vi "Revert Callback Option.vi"(11 "Callback Option String":string) -> (3 "Callback Option":T1)   [LabVIEW 2011, in "Tinkerforge.lvlib" / "Device.lvclass"]
doc: "This VI converts the Callback Option char to the callback option enumeration."
uses:
  Device.lvclass
  Type Definitions/Callback Option.ctl
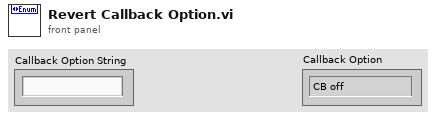
[diagram p1: front panel]
types:
  T1 = typedef "Tinkerforge.lvlib/Device.lvclass/Callback Option.ctl" = enum8{"CB off", "outside range", "inside range", "smaller", "greater"}
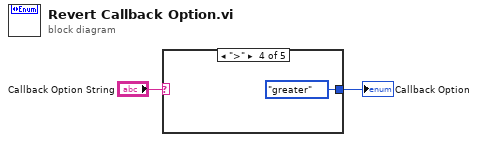
[diagram p0: block diagram]
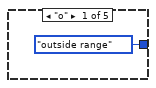
[diagram p2: hidden frame]
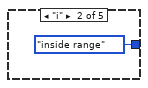
[diagram p3: hidden frame]
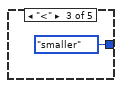
[diagram p4: hidden frame]
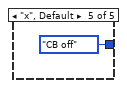
[diagram p5: hidden frame]
diagram:
  n1 = case shown="\">\"" "Callback Option String" {
    tunnel: [Callback_Option."outside range" ("Callback Option") Callback_Option."inside range" ("Callback Option") Callback_Option."smaller" ("Callback Option") Callback_Option."greater" ("Callback Option") Callback_Option."CB off" ("Callback Option")] -> w1
    frame "o" {
    }
    frame "i" {
    }
    frame "<" {
    }
    frame ">" {
    }
    frame "x", Default {
    }
  }
  "Callback Option" <- w1
